vi "SVET.vi"() -> ()   [LabVIEW 2019]
uses:
  <vilib>/LabVIEW Interface for Arduino/Type Defs/Board Type.ctl
  <vilib>/LabVIEW Interface for Arduino/Type Defs/Pin Mode.ctl
  <vilib>/LabVIEW Interface for Arduino/LabVIEW Interface for Arduino.lvlib
panel:
  in  "red":dbl(slide) scale=0.0..255.0
  in  "green":dbl(slide) scale=0.0..255.0
  in  "blue":dbl(slide) scale=0.0..255.0
  out "error out":errorcluster
  in  "Red":u8
  in  "Green":u8
  in  "Blue":u8
  in  "VISA resource":refnum<visa-resource-name>
  in  "stop":bool
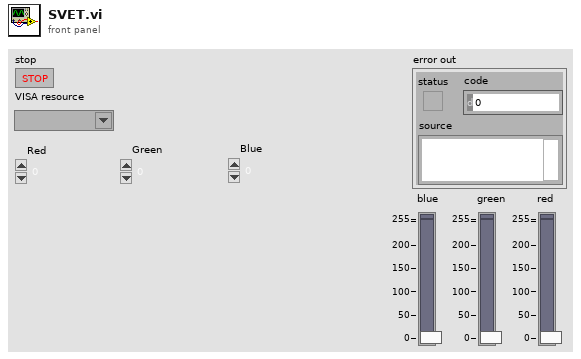
[diagram p1: front panel]
types:
  T1 = typedef "LabVIEW Interface for Arduino.lvlib/Pin Mode.ctl" = enum8{"Input", "Output"}
  T2 = typedef "LabVIEW Interface for Arduino.lvlib/Board Type.ctl" = enum16{"Uno", "Dimuelanove w/Atmega 328", "Mega 2560"}
  T3 = typedef "LabVIEW Interface for Arduino.lvlib/Arduino Resource.ctl" = cluster{"VISA resource":refnum<visa-resource-name>, "Board Type":T2, "Connection Type":enum8{"USB / Serial"}, "Bytes Per Packet (15)":u8}
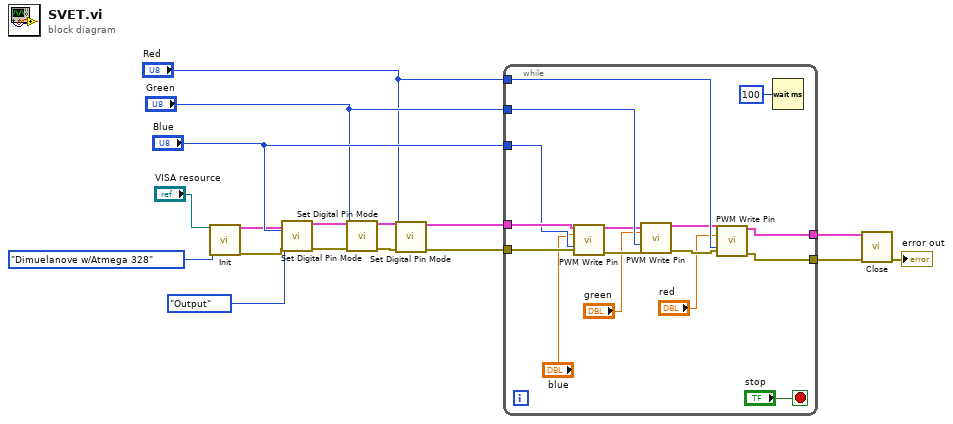
[diagram p0: block diagram]
diagram:
  n1 = call <vilib>:"Init.vi"("VISA resource"="VISA resource", "Board Type (Uno)"=Board_Type."Dimuelanove w/Atmega 328") -> ("Arduino Resource"=w1:T3, "error out"=w2:errorcluster)  [unwired: 16 in]
  n2 = call <vilib>:"Set Digital Pin Mode.vi"("Arduino Resource"=w1, "Digital I/O Pin"="Blue", "Pin Mode (Input)"=Pin_Mode."Output", "error in"=w2) -> ("Arduino Resource"=w15:T3, "error out"=w14:errorcluster)  [unwired: 10 in]
  n3 = call <vilib>:"Set Digital Pin Mode.vi"("Arduino Resource"=w15, "Digital I/O Pin"="Green", "error in"=w14) -> ("Arduino Resource"=w12:T3, "error out"=w11:errorcluster)  [unwired: 11 in]
  n4 = call <vilib>:"Set Digital Pin Mode.vi"("Arduino Resource"=w12, "Digital I/O Pin"="Red", "error in"=w11) -> ("Arduino Resource"=w10:T3, "error out"=w9:errorcluster)  [unwired: 11 in]
  n5 = while {
    tunnel: w10 -> [w31]
    tunnel: w9 -> [w30]
    tunnel: "Blue" -> [w29]
    tunnel: "Green" -> [w28]
    tunnel: "Red" -> [w27]
    tunnel: [w22] -> w5
    tunnel: [w21] -> w4
    stop <- "stop" stop-if-true
    n6 = call <vilib>:"PWM Write Pin.vi"("Arduino Resource"=w31, "Duty Cycle (0 - 255)"="blue", "PWM Pin (3)"=w29, "error in"=w30) -> ("Arduino Resource"=w26:T3, "error out"=w24:errorcluster)  [unwired: 10 in]
    n7 = call <vilib>:"PWM Write Pin.vi"("Arduino Resource"=w26, "Duty Cycle (0 - 255)"="green", "PWM Pin (3)"=w28, "error in"=w24) -> ("Arduino Resource"=w25:T3, "error out"=w23:errorcluster)  [unwired: 10 in]
    n8 = call <vilib>:"PWM Write Pin.vi"("Arduino Resource"=w25, "Duty Cycle (0 - 255)"="red", "PWM Pin (3)"=w27, "error in"=w23) -> ("Arduino Resource"=w22:T3, "error out"=w21:errorcluster)  [unwired: 10 in]
    n9 = Wait (ms)(milliseconds to wait=u32 100) -> ()  [unwired: 1 out]
  }
  n10 = call <vilib>:"Close.vi"("Arduino Resource"=w5, "error in"=w4) -> ("error out"=→"error out":errorcluster)  [unwired: 13 in]
